vi "Check Conditions.vi"(7 "Variables":refnum<class "Variables.lvclass">, 9 "Report Conditions":bool, 10 "Sequence Time":T1, 11 "Transition in":refnum<class "Transition.lvclass">) -> (1 "Met Conditions":refnum<class "Condition.lvclass">[](array[class]), 2 "Met":bool, 3 "Transition out":refnum<class "Transition.lvclass">)   [LabVIEW 2020, in "VolatusSeq.lvlib" / "Transition.lvclass"]
uses:
  Transition.lvclass
  Variables/Variables.lvclass
  Sequence Time.ctl
  Transition.lvclass/Transition.ctl
  Condition/Condition.lvclass
  VolatusSeq.lvlib
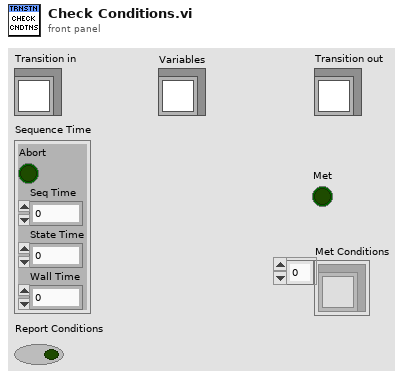
[diagram p1: front panel]
types:
  T1 = typedef "VolatusSeq.lvlib/Sequence Time.ctl" = cluster{"Abort":bool, "Seq Time":dbl, "State Time":dbl, "Wall Time":dbl}
  T2 = typedef "VolatusSeqConfig.lvlib/Condition Logic.ctl" = enum16{"All", "Any"}
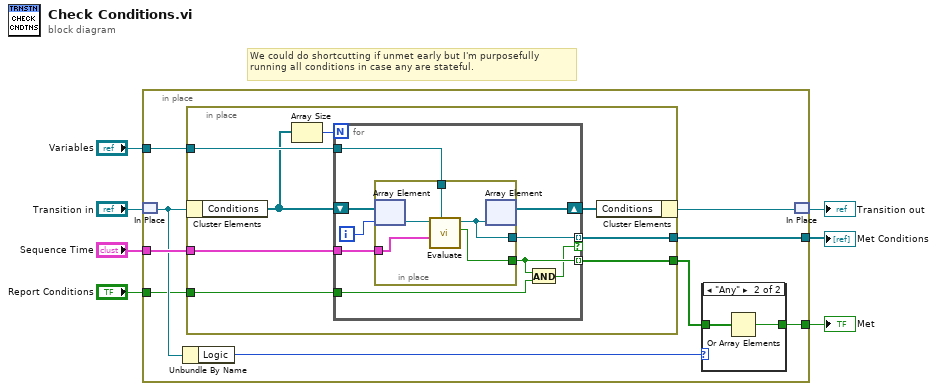
[diagram p0: block diagram]
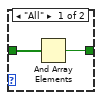
[diagram p2: hidden frame]
diagram:
  # "We could do shortcutting if unmet early but I'm purposefully running all conditions in case any are stateful."
  n1 = in-place {
    in-place-border: "Variables" -> [w15]
    in-place-border: "Sequence Time" -> [w14]
    in-place-border: [w12] -> w5
    in-place-border: "Report Conditions" -> [w9]
    in-place-border: [w8] -> w1
    n2 = in-place-match #1("Transition in") -> (w11:refnum<class "Transition.lvclass">)
    n3 = Unbundle By Name(w11) -> ("Logic"=w16:T2)
    n4 = in-place {
      in-place-border: w15 -> [w23]
      in-place-border: w14 -> [w22]
      in-place-border: [w21] -> w13
      in-place-border: w9 -> [w18]
      in-place-border: [w17] -> w8
      n5 = in-place-cluster #2(w11) -> ("Conditions"=w19:refnum<class "Condition.lvclass">[])
      n6 = Array Size(array=w19) -> (size(s)=w20:i32)
      n7 = for {
        N: w20 -> [_]
        tunnel: w23 -> [w33]
        tunnel: w22 -> [w29]
        tunnel: [w27] -> w21 mode=indexing
        shift-right: [w31] -> w24
        shift-left: w19 -> [w32]
        tunnel: w18 -> [w26]
        tunnel: [w28] -> w17 mode=indexing if=w25
        i -> [w30]
        n8 = in-place {
          in-place-border: w33 -> [w38]
          in-place-border: w29 -> [w37]
          in-place-border: [w36] -> w27
          in-place-border: [w34] -> w28
          n9 = in-place-array #3(w32, w30) -> (w35:refnum<class "Condition.lvclass">)
          n10 = call "Evaluate.vi"("Variables"=w38, "Sequence Time"=w37, "Condition in"=w35) -> ("Result"=w36:bool, "Condition out"=w34:refnum<class "Condition.lvclass">)  [unwired: 6 in, 1 out]
          n11 = in-place-array #3(w34) -> (w31:refnum<class "Condition.lvclass">[])  [unwired: 1 out]
        }
        n12 = And(x=w27, y=w26) -> (x .and. y?=w25:bool)
      }
      n13 = in-place-cluster #2("Conditions"=w24) -> (w10:refnum<class "Transition.lvclass">)
    }
    n14 = case shown="\"Any\"" w16 {
      tunnel: w13 -> [w40 w42]
      tunnel: [w39 w41] -> w12
      frame "All" {
        n15 = And Array Elements(Boolean array=w40) -> (logical AND=w39:bool)
      }
      frame "Any" {
        n16 = Or Array Elements(Boolean array=w42) -> (logical OR=w41:bool)
      }
    }
    n17 = in-place-match #1(w10) -> (→"Transition out":refnum<class "Transition.lvclass">)
  }
  "Met" <- w5
  "Met Conditions" <- w1
